vi "muestras continuas.vi"() -> ()   [LabVIEW 2016]
uses:
  <vilib>/DAQmx/write.llb/DAQmx Write (Analog 1D DBL 1Chan NSamp).vi
  <vilib>/DAQmx/create/channels.llb/DAQmx Create Channel (AO-Voltage-Basic).vi
  <vilib>/DAQmx/configure/timing.llb/DAQmx Timing (Sample Clock).vi
  <vilib>/DAQmx/miscellaneous.llb/DAQmx Fill In Error Info.vi
panel:
  in  "Stop Button":bool
  in  "Horizontal Pointer Slide":dbl(slide) scale=-25.13..25.13
  in  "Dial":dbl(knob) scale=0.0..25.13
  out "Waveform Graph":dbl[](graph)
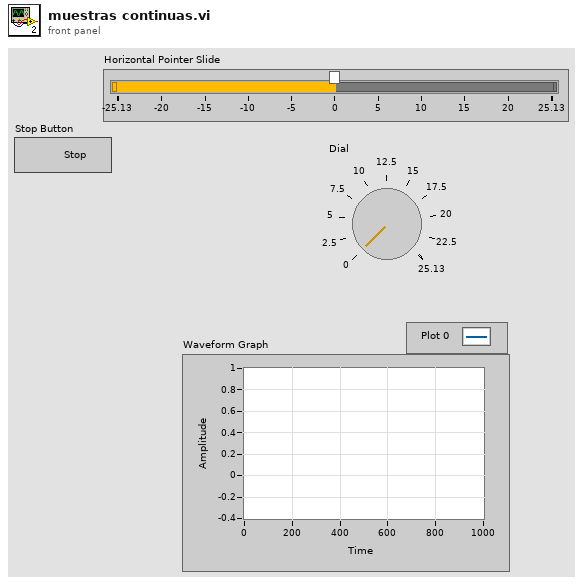
[diagram p1: front panel]
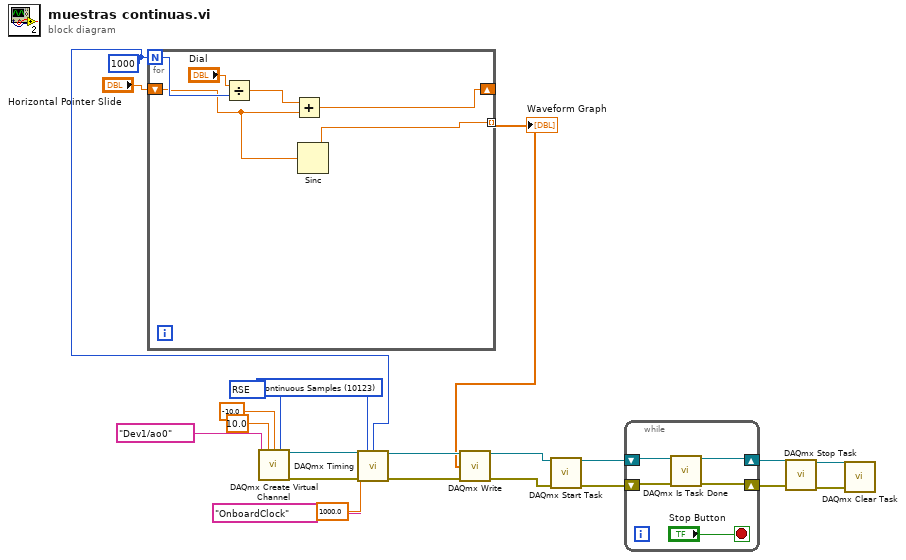
[diagram p0: block diagram]
diagram:
  w15 = 10123 items=["Finite Samples"=10178, "Continuous Samples"=10123, "Hardware Timed Single Point"=12522] ("sample mode")
  w18 = 10083 items=["Default"=-1, "RSE"=10083, "Differential"=10106, "Pseudodifferential"=12529] ("output terminal configuration")
  w14 = 1000
  n1 = for {
    N: w14 -> [w28]
    shift-right: [w26] -> _
    shift-left: "Horizontal Pointer Slide" -> [w25]
    tunnel: [w24] -> w9 mode=indexing
    n2 = Divide(x="Dial", y=w28) -> (x/y=w27:dbl)
    n3 = Add(x=w27, y=w25) -> (x+y=w26:dbl)
    n4 = Sinc(1:w25) -> (0:w24:dbl)
  }
  n5 = call-poly <vilib>:"DAQmx Create Virtual Channel.vi"("maximum value"=10.0, "minimum value"=-10.0, "output terminal configuration"=w18, "physical channels"=tag "Dev1/ao0") -> ("task out"=w17:refnum<k21>, "error out"=w16:errorcluster)  [unwired: 10 in]
  n6 = call-poly <vilib>:"DAQmx Timing.vi"("task/channels in"=w17, "sample mode"=w15, "samples per channel"=w14, "rate"=1000.0, "source"=tag "OnboardClock", "error in"=w16) -> ("task out"=w11:refnum<k21>, "error out"=w10:errorcluster)  [unwired: 8 in]
  n7 = call-poly <vilib>:"DAQmx Write.vi"("task/channels in"=w11, "data"=w9, "error in"=w10) -> ("task out"=w8:refnum<k21>, "error out"=w7:errorcluster)  [unwired: 10 in, 1 out]
  n8 = call <vilib>:"DAQmx Start Task.vi"("task/channels in"=w8, "error in"=w7) -> ("task out"=w6:refnum<k21>, "error out"=w5:errorcluster)  [unwired: 12 in]
  n9 = while {
    shift-right: [w30] -> w4
    shift-left: w6 -> [w32]
    shift-right: [w29] -> w3
    shift-left: w5 -> [w31]
    stop <- "Stop Button" stop-if-true
    n10 = call <vilib>:"DAQmx Is Task Done.vi"("task/channels in"=w32, "error in"=w31) -> ("task out"=w30:refnum<k21>, "error out"=w29:errorcluster)  [unwired: 11 in, 1 out]
  }
  n11 = call <vilib>:"DAQmx Stop Task.vi"("task/channels in"=w4, "error in"=w3) -> ("task out"=w2:refnum<k21>, "error out"=w1:errorcluster)  [unwired: 12 in]
  n12 = call <vilib>:"DAQmx Clear Task.vi"("task in"=w2, "error in"=w1) -> ()  [unwired: 13 in, 1 out]
